vi "close.vi"(8 "error in":errorcluster, 11 "MBParam in":refnum<class "TCP Param.lvclass">) -> (0 "error out":errorcluster)   [LabVIEW 2021, in "Param.lvlib" / "TCP Param.lvclass"]
uses:
  TCP Param.lvclass
  TCP Param.lvclass/TCP Param.ctl
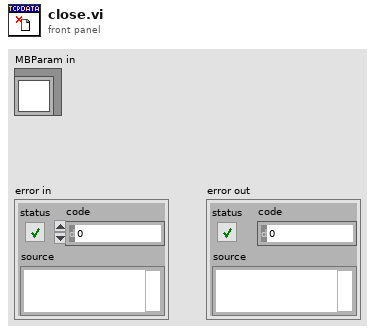
[diagram p1: front panel]
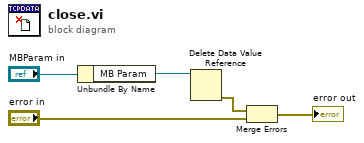
[diagram p0: block diagram]
diagram:
  n1 = Unbundle By Name("MBParam in") -> ("MB Param"=w2:refnum<data-value>)
  n2 = Delete Data Value Reference(data value reference=w2) -> (error out=w5:errorcluster)  [unwired: 1 in, 1 out]
  n3 = Merge Errors(w5, "error in") -> (→"error out":errorcluster)
